vi "Throttle Multiplier.vi"(8 "error in (no error)":errorcluster, 10 "Numeric":dbl) -> (0 "error out":errorcluster, 2 "Numeric 2":dbl)   [LabVIEW 2014]
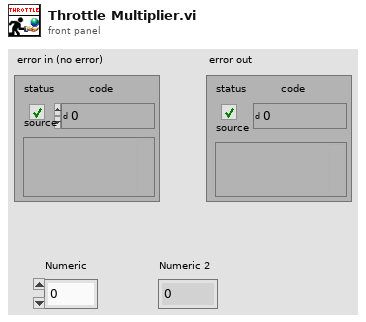
[diagram p1: front panel]
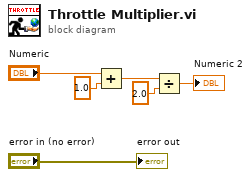
[diagram p0: block diagram]
diagram:
  n1 = Add(x="Numeric", y=1.0) -> (x+y=w4:dbl)
  n2 = Divide(x=w4, y=2.0) -> (x/y=→"Numeric 2":dbl)
  "error out" <- "error in (no error)"
